vi "servo przyklad.vi"() -> ()   [LabVIEW 2017]
uses:
  <vilib>/LabVIEW Interface for Arduino/LabVIEW Interface for Arduino.lvlib
panel:
  in  "Number of Servos":u8=2
  in  "Servo 0 Sweep Max Angle":u8=180
  out "Servo 0":dbl(knob) scale=0.0..180.0
  in  "Stop":bool
  in  "Speed":u8=1
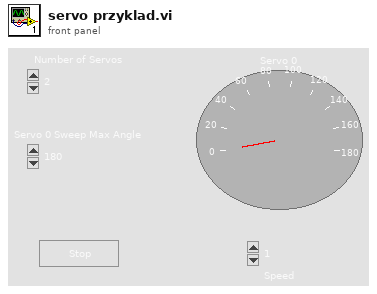
[diagram p1: front panel]
types:
  T1 = typedef "LabVIEW Interface for Arduino.lvlib/Arduino Resource.ctl" = cluster{"VISA resource":refnum<visa-resource-name>, "Board Type":T2, "Connection Type":enum8{"USB / Serial"}, "Bytes Per Packet (15)":u8}
  T2 = typedef "LabVIEW Interface for Arduino.lvlib/Board Type.ctl" = enum16{"Uno", "Dimuelanove w/Atmega 328", "Mega 2560"}
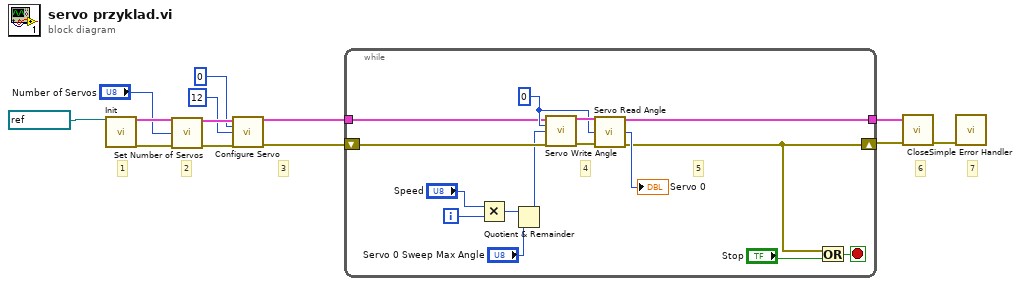
[diagram p0: block diagram]
diagram:
  # "7"
  # "6"
  # "3"
  # "2"
  # "1"
  n1 = call <vilib>:"Init.vi"("VISA resource"=refnum<visa-resource-name> "COM4") -> ("Arduino Resource"=w13:T1, "error out"=w12:errorcluster)  [unwired: 17 in]
  n2 = call <vilib>:"Set Number of Servos.vi"("Arduino Resource"=w13, "Number Of Servos (1)"="Number of Servos", "error in"=w12) -> ("Arduino Resource"=w10:T1, "error out"=w9:errorcluster)  [unwired: 11 in]
  n3 = call <vilib>:"Configure Servo.vi"("Arduino Resource"=w10, "Servo Number (0)"=u8 0 ("Servo Number"), "DIO Pin (2)"=u8 12 ("Servo Number"), "error in"=w9) -> ("Arduino Resource"=w2:T1, "error out"=w3:errorcluster)  [unwired: 10 in]
  n4 = while {
    shift-right: [w14] -> w6
    shift-left: w3 -> [w27]
    tunnel: w2 -> [w16]
    tunnel: [w15] -> w1
    i -> [w18]
    stop <- w23 stop-if-true
    w22 = u8 0 ("Servo Number")
    # "5"
    # "4"
    n5 = Multiply(x="Speed", y=w18) -> (x*y=w19:i32)
    n6 = Quotient & Remainder(x=w19, y="Servo 0 Sweep Max Angle") -> (x-y*floor(x/y)=w25:i32)  [unwired: 1 out]
    n7 = call <vilib>:"Servo Write Angle.vi"("Arduino Resource"=w16, "Servo Number"=w22, "Angle (Degrees)"=w25, "error in"=w27) -> ("Arduino Resource"=w28:T1, "error out"=w26:errorcluster)  [unwired: 10 in]
    n8 = call <vilib>:"Servo Read Angle.vi"("Arduino Resource"=w28, "Servo Number"=w22, "error in"=w26) -> ("Arduino Resource"=w15:T1, "Angle (Degrees)"=→"Servo 0":u8, "error out"=w14:errorcluster)  [unwired: 10 in]
    n9 = Or(x=w14, y="Stop") -> (x .or. y?=w23:bool)
  }
  n10 = call <vilib>:"Close.vi"("Arduino Resource"=w1, "error in"=w6) -> ("error out"=w4:errorcluster)  [unwired: 13 in]
  n11 = call <vilib>:"Simple Error Handler.vi"("error in (no error)"=w4) -> ()  [unwired: 4 in, 5 out]
